vi "Generate simulated control timings sequence.vi"(7 "ROI Dwell time":dbl, 9 "High value of simulated waveform":dbl, 10 "Time resolution of simulated waveform":dbl, 11 "Number of POI":i32) -> (3 "Simulated control timings sequence in":waveform(dbl))   [LabVIEW 2020]
uses:
  Global Variables/General Globals.vi
  <vilib>/Waveform/WDTOps.llb/WDT Append Waveforms DBL.vi
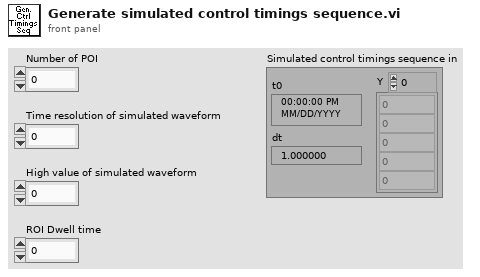
[diagram p1: front panel]
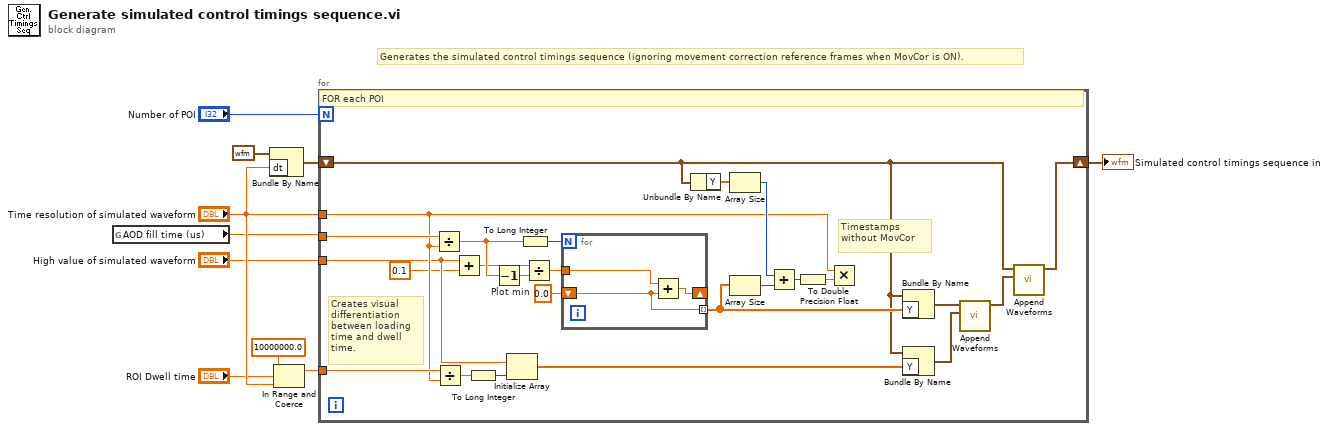
[diagram p0: block diagram]
diagram:
  # "Generates the simulated control timings sequence (ignoring movement correction reference frames when MovCor is ON)."
  n1 = global read "General Globals.vi" "AOD fill time (us)"() -> (w6:dbl)
  n2 = Bundle By Name ("Build Waveform")(cluster=waveform(dbl) {"t0"=timestamp(0 s since 1904-01-01), "dt"=0.0, "Y"=[]} ("waveform out"), "dt"="Time resolution of simulated waveform") -> (w1:waveform(dbl))
  n3 = In Range and Coerce(upper limit=10000000.0, x="ROI Dwell time", lower limit="Time resolution of simulated waveform") -> (coerced(x)=w4:dbl)  [unwired: 1 out]
  n4 = for {
    N: "Number of POI" -> [_]
    shift-right: [w28] -> w7
    shift-left: w1 -> [w14]
    tunnel: "Time resolution of simulated waveform" -> [w15]
    tunnel: w4 -> [w23]
    tunnel: w6 -> [w22]
    tunnel: "High value of simulated waveform" -> [w13]
    w35 = 0.0  # Plot min
    # "Creates visual differentiation between loading time and dwell time."
    # "Timestamps without MovCor"
    # "FOR each POI"
    n5 = Divide(x=w22, y=w15) -> (x/y=w25:dbl)
    n6 = Divide(x=w23, y=w15) -> (x/y=w33:dbl)
    n7 = Add(x=w13, y=0.1) -> (x+y=w12:dbl)
    n8 = To Long Integer(number=w33) -> (32bit integer=w32:i32)
    n9 = Decrement(x=w25) -> (x-1=w24:dbl)
    n10 = Initialize Array(w13, w32) -> (w31:dbl[])
    n11 = To Long Integer(number=w25) -> (32bit integer=w26:i32)
    n12 = Divide(x=w12, y=w24) -> (x/y=w34:dbl)
    n13 = for {
      N: w26 -> [_]
      shift-right: [w37] -> _
      shift-left: w35 -> [w36]
      tunnel: w34 -> [w38]
      tunnel: [w36] -> w20 mode=indexing
      n14 = Add(x=w38, y=w36) -> (x+y=w37:dbl)
    }
    n15 = Unbundle By Name(w14) -> ("Y"=w21:dbl[])
    n16 = Array Size(array=w21) -> (size(s)=w19:i32)
    n17 = Array Size(array=w20) -> (size(s)=w18:i32)
    n18 = Add(x=w19, y=w18) -> (x+y=w17:i32)
    n19 = To Double Precision Float(number=w17) -> (double precision float=w16:dbl)
    n20 = Multiply(x=w15, y=w16) -> ()  [unwired: 1 out]
    n21 = Bundle By Name(cluster=w14, "Y"=w20) -> (w30:waveform(dbl))
    n22 = Bundle By Name(cluster=w14, "Y"=w31) -> (w29:waveform(dbl))
    n23 = call-poly <vilib>:"Append Waveforms.vi"("waveform B"=w29, "waveform A"=w30) -> ("waveform out"=w27:waveform(dbl))  [unwired: 8 in, 1 out]
    n24 = call-poly <vilib>:"Append Waveforms.vi"("waveform B"=w27, "waveform A"=w14) -> ("waveform out"=w28:waveform(dbl))  [unwired: 8 in, 1 out]
  }
  "Simulated control timings sequence in" <- w7
